vi "Advance past next JSON Value.vi"(7 "JSON":string, 9 "Offset":i32) -> (1 "Offset out":i32, 2 "Value start":i32, 3 "State":T1=enum."Value end")   [LabVIEW 2024, in "JSONtext.lvlib"]
uses:
  JSONtext.lvlib
  Parsing State.ctl
  Advance past Line Ending.vi
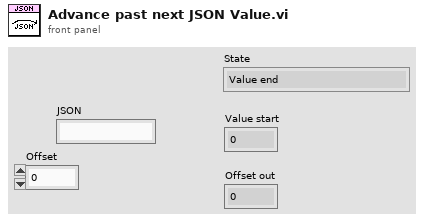
[diagram p1: front panel]
types:
  T1 = typedef "JSONtext.lvlib/Parsing State.ctl" = enum16{"Parser Error", "Object", "Array", "String", "Number/Other", "Leading Whitespace", "Object end", "Array end", "Value end"}
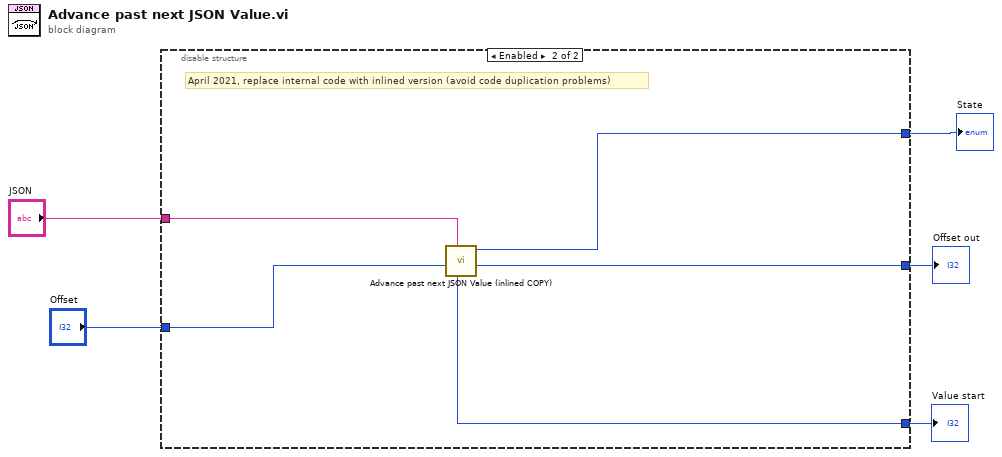
[diagram p0: block diagram]
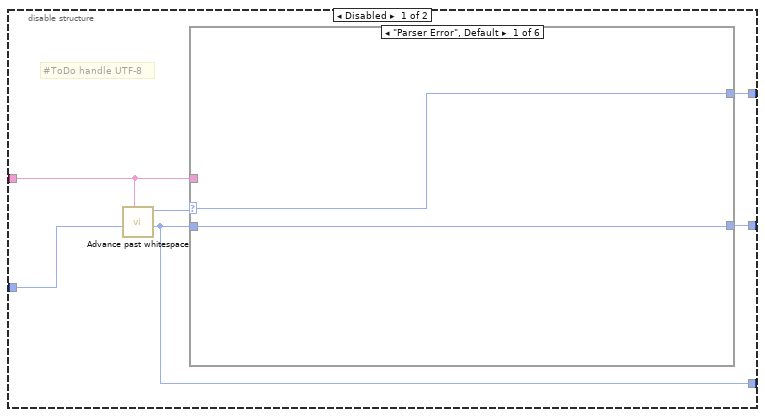
[diagram p2: hidden frame]
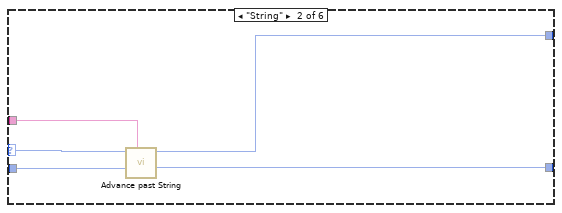
[diagram p3: hidden frame]
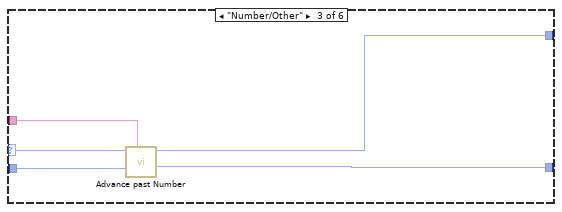
[diagram p4: hidden frame]
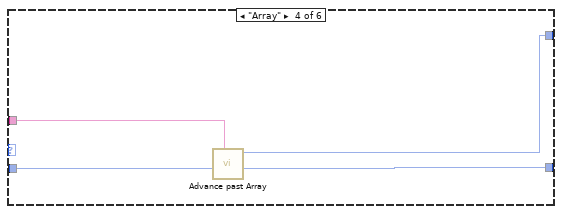
[diagram p5: hidden frame]
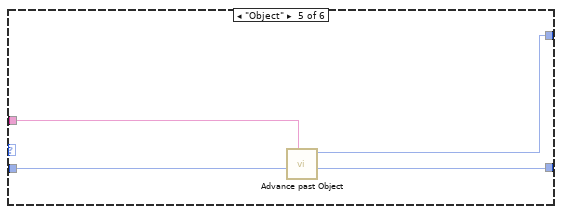
[diagram p6: hidden frame]
diagram:
  n1 = disable-structure shown="Enabled" {
    disable-tunnel: "JSON" -> [w11 w38]
    disable-tunnel: [w9 w35] -> w4
    disable-tunnel: [w8 w36] -> w3
    disable-tunnel: "Offset" -> [w7 w37]
    disable-tunnel: [w6 w34] -> w1
    frame Disabled {
      # "#ToDo handle UTF-8"
      n2 = call "Advance past whitespace.vi"("JSON"=w11, "Offset"=w7) -> ("Offset of first non-whitespace"=w6:i32, "Parser State"=w10:T1)  [unwired: 7 in, 1 out]
      n3 = case shown="\"Parser Error\", Default" w10 {
        selector: w10 -> [w12 w17 w22 _ _ w32]
        tunnel: w11 -> [_ w18 w23 w24 w28 _]
        tunnel: w6 -> [w13 w16 w21 w25 w31 w33]
        tunnel: [w13 w15 w20 w26 w29 w33] -> w9
        tunnel: [w12 w14 w19 w27 w30 w32] -> w8
        frame "Parser Error", Default {
        }
        frame "String" {
          n4 = call "Advance past String.vi"("JSON"=w18, "Offset"=w16, "State in"=w17) -> ("Offset past match"=w15:i32, "State"=w14:T1)  [unwired: 6 in, 1 out]
        }
        frame "Number/Other" {
          n5 = call "Advance past Number.vi"("JSON"=w23, "Offset (0)"=w21, "Parser State in"=w22) -> ("Offset past match"=w20:i32, "Parser State"=w19:T1)  [unwired: 4 in, 3 out]
        }
        frame "Array" {
          n6 = call "Advance past Array.vi"("JSON"=w24, "Offset"=w25) -> ("Offset past Array"=w26:i32, "State"=w27:T1)  [unwired: 6 in, 2 out]
        }
        frame "Object" {
          n7 = call "Advance past Object.vi"("JSON"=w28, "Offset"=w31) -> ("Offset past Object"=w29:i32, "State"=w30:T1)  [unwired: 7 in, 1 out]
        }
        frame "Value end" {
          # "null, true, etc."
        }
      }
    }
    frame Enabled {
      # "April 2021, replace internal code with inlined version (avoid code duplication problems)"
      n8 = call "Advance past next JSON Value (inlined COPY).vi"("JSON"=w38, "Offset"=w37) -> ("Offset"=w35:i32, "State"=w36:T1, "Value start"=w34:i32)  [unwired: 5 in, 2 out]
    }
  }
  "State" <- w3
  "Offset out" <- w4
  "Value start" <- w1
